vi "GT Crd Data Circle.vi"(7 "fifo":i16, 8 "error in (no error)":errorcluster caption="错误输入（无错误）", 9 "pCrdData":T1, 10 "crd":i16, 11 "cardNum":i16) -> (0 "error out":errorcluster caption="错误输出", 1 "pCrdData out":T1, 3 "function return":i16)   [LabVIEW 2014, in "gts.lvlib"]
doc: "GT_API GT_CrdDataCircle(short cardNum,short crd,TCrdData *pCrdData,short fifo=0);"
uses:
  gts.lvlib
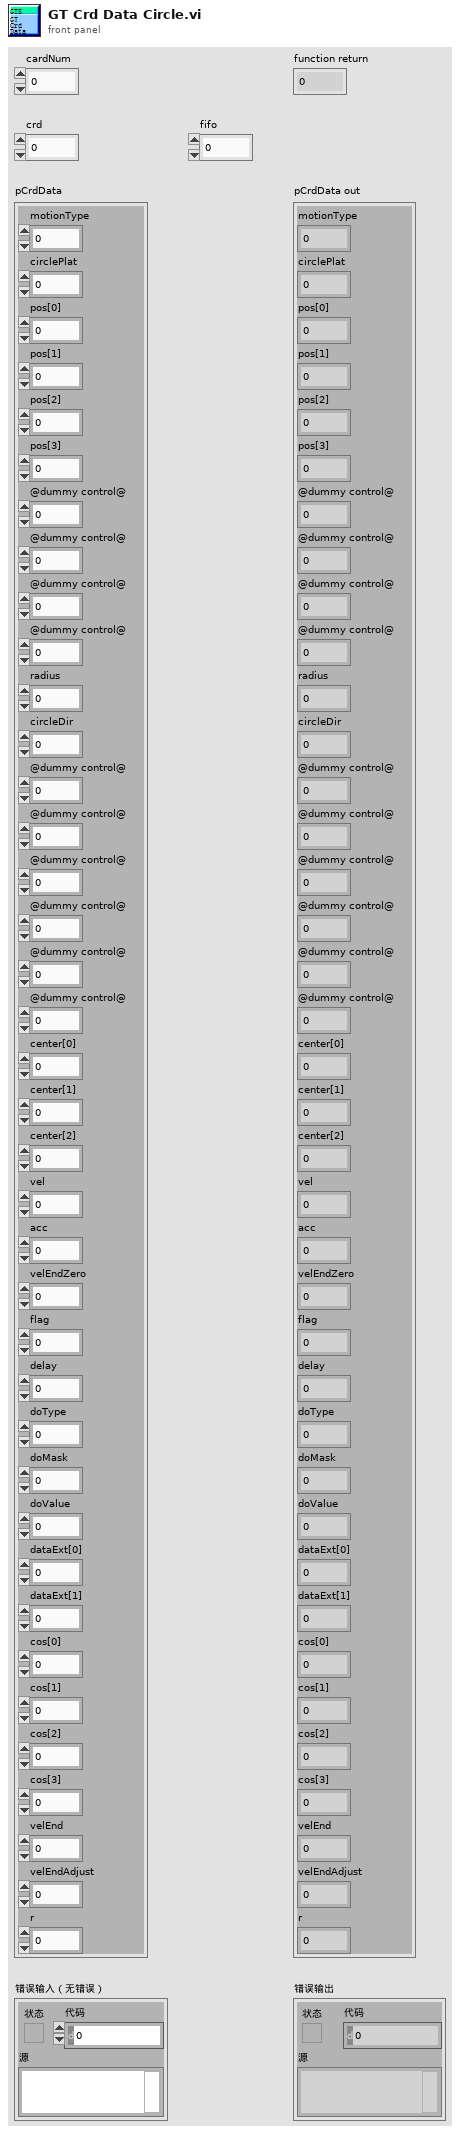
[diagram p1: front panel]
types:
  T1 = cluster{"motionType":i16, "circlePlat":i16, "pos[0]":i32, "pos[1]":i32, "pos[2]":i32, "pos[3]":i32, "@dummy control@":i8, "@dummy control@":i8, "@dummy control@":i8, "@dummy control@":i8, "radius":dbl, "circleDir":i16, "@dummy control@":i8, "@dummy control@":i8, "@dummy control@":i8, "@dummy control@":i8, "@dummy control@":i8, "@dummy control@":i8, "center[0]":dbl, "center[1]":dbl, "center[2]":dbl, "vel":dbl, "acc":dbl, "velEndZero":i16, "flag":i16, "delay":u16, "doType":i16, "doMask":u16, "doValue":u16, "dataExt[0]":u16, "dataExt[1]":u16, "cos[0]":dbl, "cos[1]":dbl, "cos[2]":dbl, "cos[3]":dbl, "velEnd":dbl, "velEndAdjust":dbl, "r":dbl}
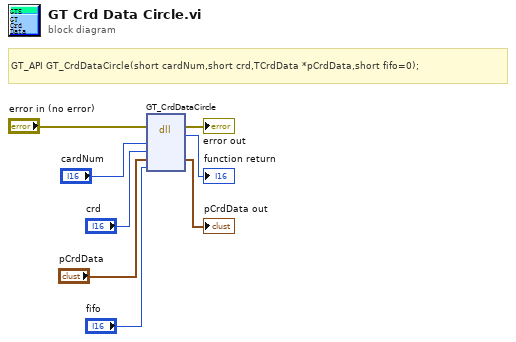
[diagram p0: block diagram]
diagram:
  # "GT_API GT_CrdDataCircle(short cardNum,short crd,TCrdData *pCrdData,short fifo=0);"
  n1 = dll-call lib="PTH2habs D固高科技资料GTS控制卡GTS卡18年上半年资料dllVC32bit\nmulti_cardgts.*" fn="GT_CrdDataCircle"(error in="error in (no error)", "cardNum"="cardNum", "crd"="crd", "pCrdData"="pCrdData", "fifo"="fifo") -> (error out=→"error out":errorcluster, →"function return":i16, "pCrdData"=→"pCrdData out":T1)  [unwired: 5 in, 1 out]
